vi "Read Controller Actor Enqueuer.vi"(8 "error in (no error)":errorcluster, 11 "View Actor in":refnum<class "View Actor.lvclass">) -> (0 "error out":errorcluster, 2 "Controller Actor Enqueuer":refnum<class "Message Enqueuer.lvclass">, 3 "View Actor out":refnum<class "View Actor.lvclass">)   [LabVIEW 2016, in "Event Actors.lvlib" / "View Actor.lvclass"]
uses:
  View Actor.lvclass
  <vilib>/ActorFramework/Message Enqueuer/Message Enqueuer.lvclass
  View Actor.lvclass/View Actor.ctl
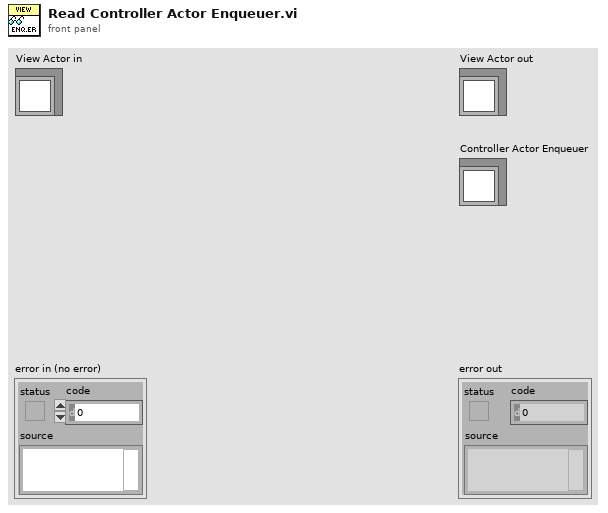
[diagram p1: front panel]
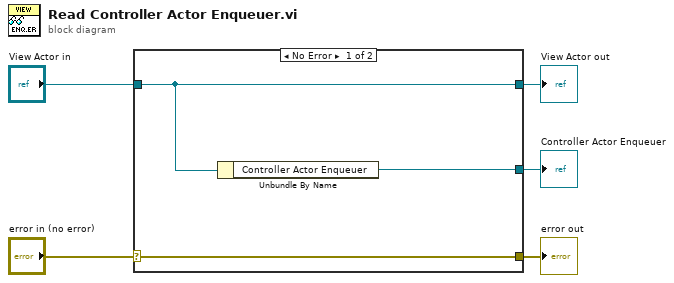
[diagram p0: block diagram]
diagram:
  n1 = case shown="No Error" "error in (no error)" {
    selector: "error in (no error)" -> [w8 w9]
    tunnel: [w8 w9] -> w4
    tunnel: [w7 w10] -> w2
    tunnel: "View Actor in" -> [w7 w10]
    tunnel: [w6 _] -> w1
    frame No Error {
      n2 = Unbundle By Name(w7) -> ("Controller Actor Enqueuer"=w6:refnum<class "Message Enqueuer.lvclass">)
    }
    frame Error {
    }
  }
  "error out" <- w4
  "View Actor out" <- w2
  "Controller Actor Enqueuer" <- w1
